vi "piezoDoubleWriteOpen.vi"() -> ()   [LabVIEW 2017]
uses:
  <vilib>/DAQmx/write.llb/DAQmx Write (Analog 2D DBL NChan NSamp).vi
  <vilib>/DAQmx/write.llb/DAQmx Write (Analog 1D DBL NChan 1Samp).vi
  globalDevices.vi
  <vilib>/DAQmx/create/channels.llb/DAQmx Create Channel (AO-Voltage-Basic).vi
  <vilib>/DAQmx/configure/timing.llb/DAQmx Timing (Sample Clock).vi
  <vilib>/DAQmx/miscellaneous.llb/DAQmx Fill In Error Info.vi
  Piezo/lvlib/Madlib.lvlib
panel:
  out "Waveform Graph":dbl[](graph)
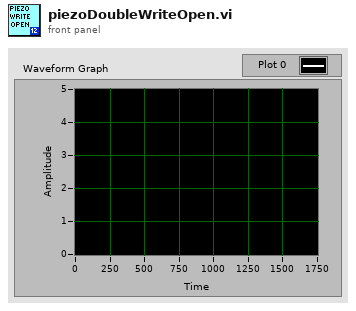
[diagram p1: front panel]
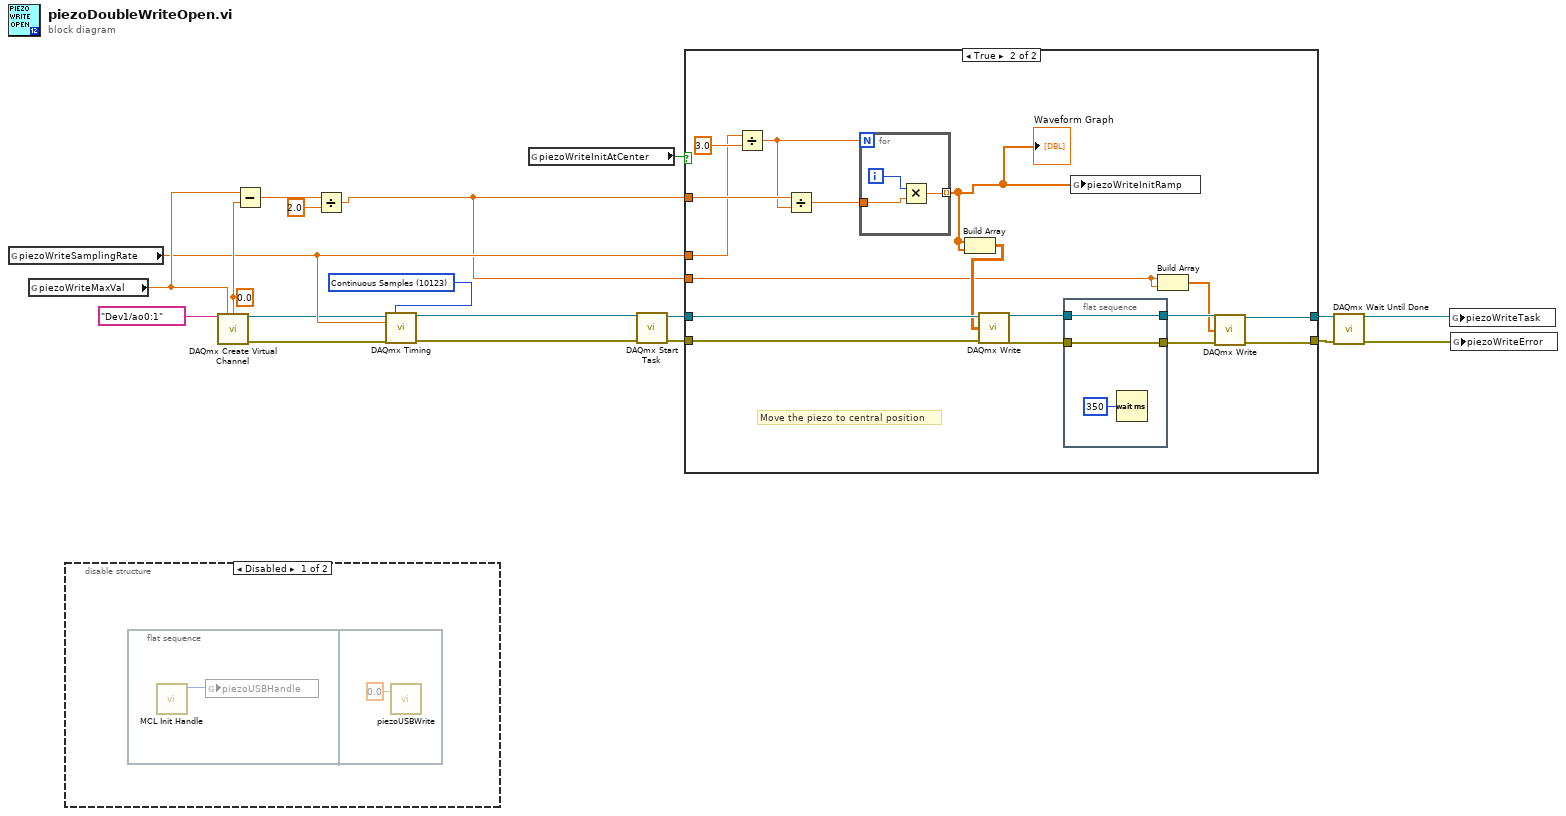
[diagram p0: block diagram]
diagram:
  w15 = 10123 items=["Finite Samples"=10178, "Continuous Samples"=10123, "Hardware Timed Single Point"=12522] ("sample mode")
  w18 = 0.0 ("minimum value")
  n1 = global read "globalDevices.vi" "piezoWriteSamplingRate"() -> (w16:dbl)
  n2 = global read "globalDevices.vi" "piezoWriteMaxVal"() -> (w19:dbl)
  n3 = disable-structure shown="Disabled" {
    frame Disabled {
      n4 = flat-sequence {
        frame #0 {
          n5 = call "MCL Init Handle.vi"() -> ("function return"=w20:i32)  [unwired: 11 in]
          n6 = global write "globalDevices.vi" "piezoUSBHandle"(w20) -> ()
        }
        frame #1 {
          n7 = call "piezoUSBWrite.vi"("position"=0.0) -> ()  [unwired: 2 in]
        }
      }
    }
    frame Enabled {
    }
  }
  n8 = call-poly <vilib>:"DAQmx Create Virtual Channel.vi"("maximum value"=w19, "minimum value"=w18, "physical channels"=tag "Dev1/ao0:1") -> ("task out"=w14:refnum<k21>, "error out"=w13:errorcluster)  [unwired: 11 in]
  n9 = Subtract(x=w19, y=w18) -> (x-y=w17:dbl)
  n10 = Divide(x=w17, y=2.0) -> (x/y=w11:dbl)
  n11 = call-poly <vilib>:"DAQmx Timing.vi"("task/channels in"=w14, "sample mode"=w15, "rate"=w16, "error in"=w13) -> ("task out"=w10:refnum<k21>, "error out"=w9:errorcluster)  [unwired: 10 in]
  n12 = global read "globalDevices.vi" "piezoWriteInitAtCenter"() -> (w6:bool)
  n13 = call <vilib>:"DAQmx Start Task.vi"("task/channels in"=w10, "error in"=w9) -> ("task out"=w7:refnum<k21>, "error out"=w8:errorcluster)  [unwired: 12 in]
  n14 = case shown="True" w6 {
    tunnel: w7 -> [w23 w34]
    tunnel: w8 -> [w22 w35]
    tunnel: w11 -> [_ w39]
    tunnel: w16 -> [_ w36]
    tunnel: [w23 w33] -> w3
    tunnel: [w22 w32] -> w4
    tunnel: w11 -> [_ w25]
    frame False {
    }
    frame True {
      # "Move the piezo to central position"
      n15 = Divide(x=w36, y=3.0) -> (x/y=w38:dbl)
      n16 = Divide(x=w39, y=w38) -> (x/y=w37:dbl)
      n17 = for {
        N: w38 -> [_]
        tunnel: w37 -> [w45]
        tunnel: [w44] -> w27 mode=indexing
        i -> [w46]
        n18 = Multiply(x=w46, y=w45) -> (x*y=w44:dbl)
      }
      "Waveform Graph" <- w27
      n19 = Build Array(w27, w27) -> (w26:dbl[][])
      n20 = call-poly <vilib>:"DAQmx Write.vi"("task/channels in"=w34, "data"=w26, "error in"=w35) -> ("task out"=w31:refnum<k21>, "error out"=w28:errorcluster)  [unwired: 10 in, 1 out]
      n21 = flat-sequence {
        tunnel: w31 -> [w43]
        tunnel: [w43] -> w30
        tunnel: [w42] -> w29
        tunnel: w28 -> [w42]
        frame #0 {
          n22 = Wait (ms)(milliseconds to wait=u32 350) -> ()  [unwired: 1 out]
        }
      }
      n23 = global write "globalDevices.vi" "piezoWriteInitRamp"(w27) -> ()
      n24 = Build Array(w25, w25) -> (w24:dbl[])
      n25 = call-poly <vilib>:"DAQmx Write.vi"("task/channels in"=w30, "data"=w24, "error in"=w29) -> ("task out"=w33:refnum<k21>, "error out"=w32:errorcluster)  [unwired: 10 in, 1 out]
    }
  }
  n26 = call <vilib>:"DAQmx Wait Until Done.vi"("task/channels in"=w3, "error in"=w4) -> ("task out"=w2:refnum<k21>, "error out"=w1:errorcluster)  [unwired: 12 in]
  n27 = global write "globalDevices.vi" "piezoWriteTask"(w2) -> ()
  n28 = global write "globalDevices.vi" "piezoWriteError"(w1) -> ()
